vi "formatIntoRowInterface.vi"(8 "error in (no error)":errorcluster, 11 "Category in":refnum<class "Category.lvclass">) -> (0 "error out":errorcluster, 2 "Row Interface":string[](array[string]), 3 "Category out":refnum<class "Category.lvclass">)   [LabVIEW 2018, in "Category.lvclass"]
uses:
  Category.lvclass
  C:/GitRepos/Filthy-Lucre-Budgetizer/source/support/classes/UserEditableAmount/UserEditableAmount.lvclass
  Category.lvclass/Category.ctl
  UserEditableAmount/UserEditableAmount.lvclass
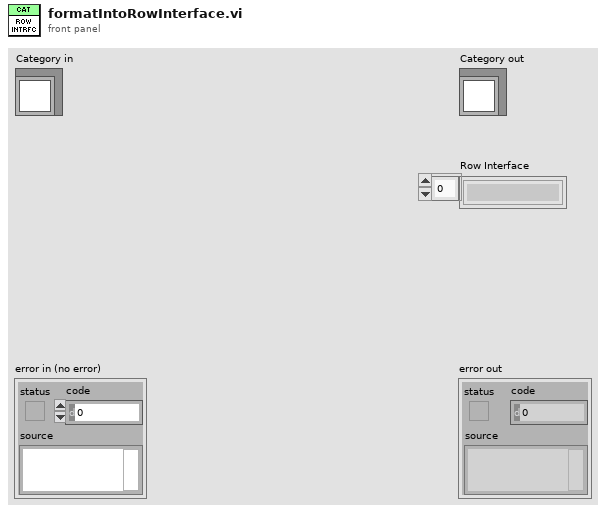
[diagram p1: front panel]
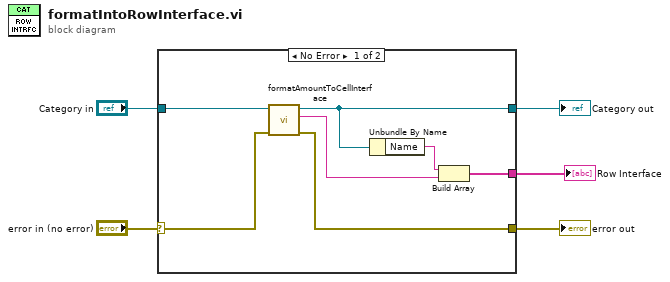
[diagram p0: block diagram]
diagram:
  n1 = case shown="No Error" "error in (no error)" {
    selector: "error in (no error)" -> [w12 w14]
    tunnel: [w11 w14] -> w4
    tunnel: [w9 w13] -> w2
    tunnel: "Category in" -> [w10 w13]
    tunnel: [w6 _] -> w1
    frame No Error {
      n2 = call "formatAmountToCellInterface.vi"("error in (no error)"=w12, "UserEditableAmount in"=w10) -> ("error out"=w11:errorcluster, "Cell Interface"=w7:string, "UserEditableAmount out"=w9:refnum<class "Category.lvclass">)  [unwired: 7 in]
      n3 = Unbundle By Name(w9) -> ("Name"=w8:string)
      n4 = Build Array(w8, w7) -> (w6:string[])
    }
    frame Error {
    }
  }
  "error out" <- w4
  "Category out" <- w2
  "Row Interface" <- w1
